vi "4Pi Capture Set Auto Waveform.vi"(0 "Interline Interval":dbl, 11 "Waveform Parameters":dbl[](array[numeric])) -> (4 "Offset (V)":dbl, 6 "Amplitude (V)":dbl, 8 "Samples per Channel":i32, 10 "Delay (ms)":dbl, 13 "Line Scan Settings":T1)   [LabVIEW 2021]
uses:
  4Pi Capture Manager Controls/4Pi Capture Line Scan Settings.ctl
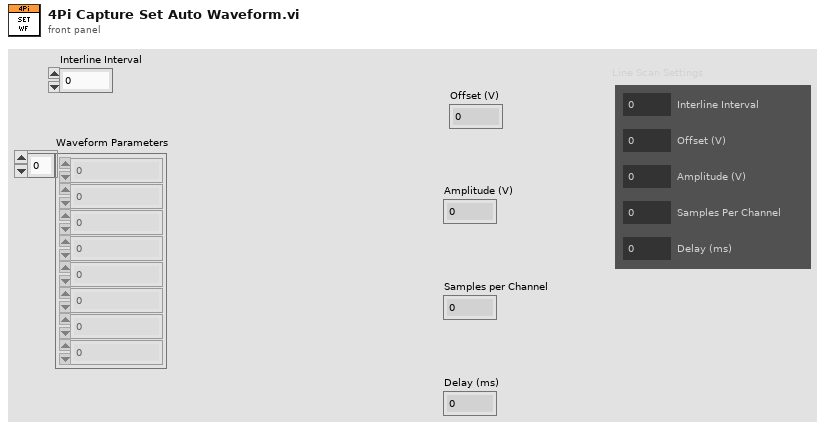
[diagram p1: front panel]
types:
  T1 = typedef "4Pi Capture Line Scan Settings.ctl" = cluster{"Interline Interval":dbl, "Offset (V)":dbl, "Amplitude (V)":dbl, "Samples Per Channel":dbl, "Delay (ms)":dbl}
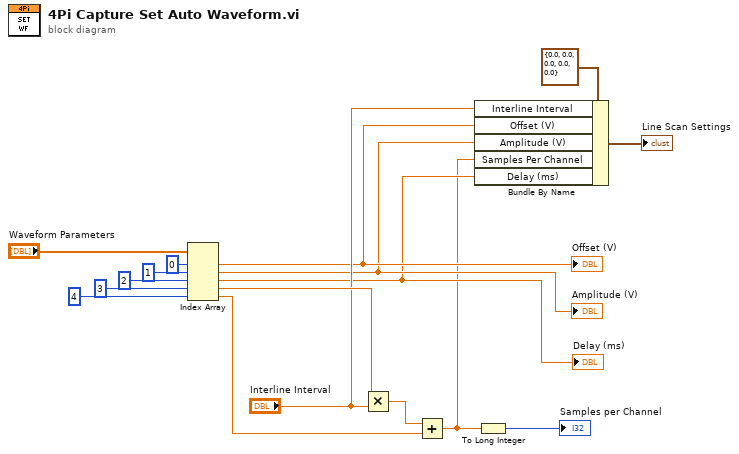
[diagram p0: block diagram]
diagram:
  n1 = Index Array(array="Waveform Parameters", index #1=0 ("index"), index #2=1 ("index"), index #3=2 ("index"), index #4=3 ("index"), index #5=4 ("index")) -> (element #1=w5:dbl, element #2=w4:dbl, element #3=w3:dbl, element #4=w11:dbl, element #5=w9:dbl)
  "Offset (V)" <- w5
  "Amplitude (V)" <- w4
  "Delay (ms)" <- w3
  n2 = Multiply(x=w11, y="Interline Interval") -> (x*y=w10:dbl)
  n3 = Add(x=w10, y=w9) -> (x+y=w2:dbl)
  n4 = Bundle By Name(cluster=T1 {"Interline Interval"=0.0, "Offset (V)"=0.0, "Amplitude (V)"=0.0, "Samples Per Channel"=0.0, "Delay (ms)"=0.0} ("Line Scan Settings"), "Interline Interval"="Interline Interval", "Offset (V)"=w5, "Amplitude (V)"=w4, "Samples Per Channel"=w2, "Delay (ms)"=w3) -> (→"Line Scan Settings":T1)
  n5 = To Long Integer(number=w2) -> (32bit integer=→"Samples per Channel":i32)
